vi "to_json.vi"(8 "error in":errorcluster, 11 "scaleParameter in":refnum<class "scaleParameter.lvclass">) -> (0 "error out":errorcluster, 2 "json":string, 3 "scaleParameter out":refnum<class "scaleParameter.lvclass">, 4 "Not Default":bool)   [LabVIEW 2020, in "nominal types.lvlib" / "timestampManifest.lvlib" / "scaleParameter.lvclass"]
uses:
  scaleParameter.lvclass
  scaleParameter.lvclass/scaleParameter.ctl
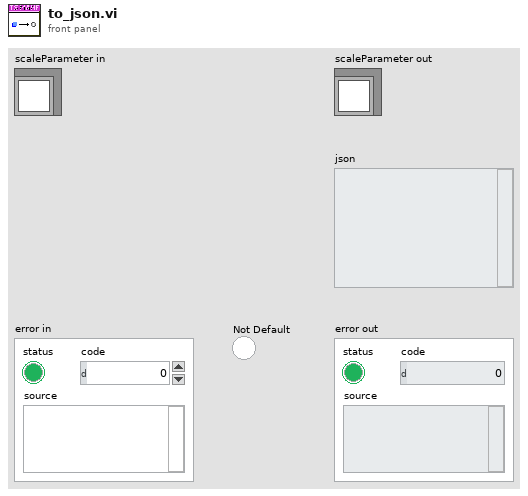
[diagram p1: front panel]
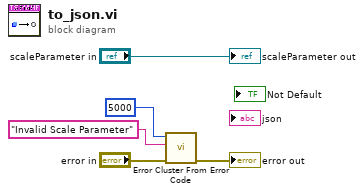
[diagram p0: block diagram]
diagram:
  n1 = call <vilib>:"Error Cluster From Error Code.vi"("error in (no error)"="error in", "error message (\"\")"="Invalid Scale Parameter" ("error message (\"\")"), "error code (0)"=5000) -> ("error out"=→"error out":errorcluster)  [unwired: 6 in]
  "scaleParameter out" <- "scaleParameter in"
